vi "Get Serial Channel I2C Name.vi"(8 "error in (no error)":errorcluster, 10 "Serial Channel":string, 11 "FGPA Ref in":refnum<k20>) -> (0 "error out":errorcluster, 2 "SO/SI I2C Name":string, 3 "FPGA Ref out":refnum<k20>)   [LabVIEW 2025, in "I2C Bus Monitor.lvclass"]
uses:
  I2C Bus Monitor.lvclass
  <instrlib>/FlexRIO/API/Host/v1/NI FlexRIO/API/Get Property Reference - Fpga Small.vi
  <resource>/objmgr/niflexrioapiChannel.rc
  <instrlib>/FlexRIO/API/Host/v1/NI FlexRIO API v1.lvlib
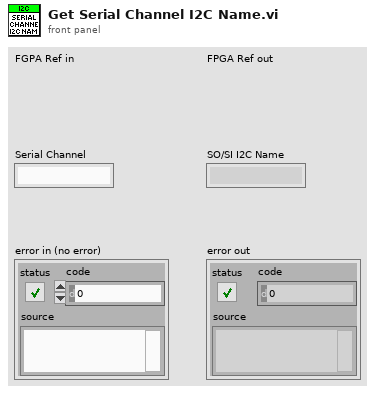
[diagram p1: front panel]
types:
  T1 = enum16{"Serial Input Channel", "Serial Output Channel", "Unknown Channel Type"}
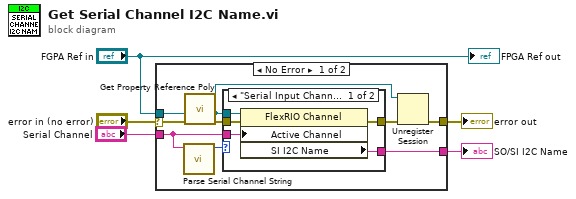
[diagram p0: block diagram]
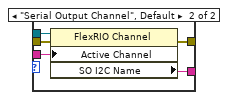
[diagram p2: hidden frame]
diagram:
  n1 = case shown="No Error" "error in (no error)" {
    selector: "error in (no error)" -> [w7 w25]
    tunnel: [w13 w25] -> w5
    tunnel: "Serial Channel" -> [w11 _]
    tunnel: [w10 _] -> w3
    tunnel: "FGPA Ref in" -> [w6 _]
    frame No Error {
      n2 = call "Parse Serial Channel String.vi"("Serial Channel String"=w11) -> ("Serial Channel Type"=w8:T1)  [unwired: 9 in, 1 out]
      n3 = call-poly <instrlib>:"Get Property Reference Poly.vi"("error in (no error)"=w7, "fpga interface in"=w6) -> ("error out"=w9:errorcluster, "property reference"=w14:refnum<k20>)  [unwired: 4 in, 1 out]
      n4 = case shown="\"Serial Input Channel\"" w8 {
        tunnel: [w19 w24] -> w10
        tunnel: [w15 w23] -> w12
        tunnel: w9 -> [w18 w22]
        tunnel: w14 -> [w17 w21]
        tunnel: w11 -> [w16 w20]
        frame "Serial Input Channel" {
          n5 = property class="FlexRIO Channel"(reference=w17, error in=w18, "Active Channel"=w16) -> (error out=w15:errorcluster, "SI I2C Name"=w19:string)  [unwired: 1 out]
        }
        frame "Serial Output Channel", Default {
          n6 = property class="FlexRIO Channel"(reference=w21, error in=w22, "Active Channel"=w20) -> (error out=w23:errorcluster, "SO I2C Name"=w24:string)  [unwired: 1 out]
        }
      }
      n7 = Unregister Session(8:w12, 11:w14) -> (0:w13:errorcluster)
    }
    frame Error {
    }
  }
  "error out" <- w5
  "SO/SI I2C Name" <- w3
  "FPGA Ref out" <- "FGPA Ref in"
